vi "Test_ANN.vi"(8 "error in (no error)":errorcluster, 11 "FPGA VI Reference In":refnum<k20>) -> (0 "error out":errorcluster, 2 "Acc":dbl, 3 "FPGA VI Reference Out":refnum<k20>)   [LabVIEW 2020]
uses:
  <vilib>/Utility/error.llb/Error Cluster From Error Code.vi
  <vilib>/rvi/errors/niLvFpgaAdjustHostInterfaceError.vi
  Store Training and Testing set.vi
  <vilib>/rvi/interface/nirviMethod/nirviMethod.xnode
  <vilib>/FPGAPlugInAG/Dynamic/niLvFpga_WriteFifo_Dynamic.vi
  <vilib>/rvi/errors/niLvFpgaMergeErrorWithErrorCode.vi
  <vilib>/FPGAPlugInAG/Dynamic/niLvFpga_ReadFifo_Dynamic.vi
panel:
  out "Prediction":sgl[](array[numeric])
  out "Real":sgl[](array[numeric])
  out "good":i32
  out "total":i32
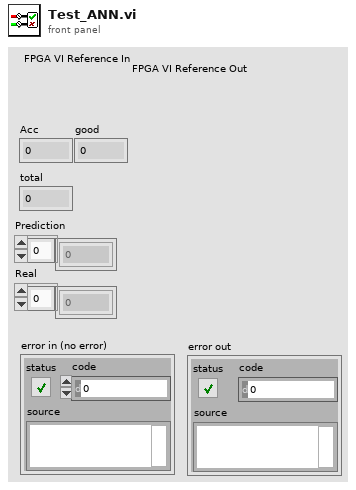
[diagram p1: front panel]
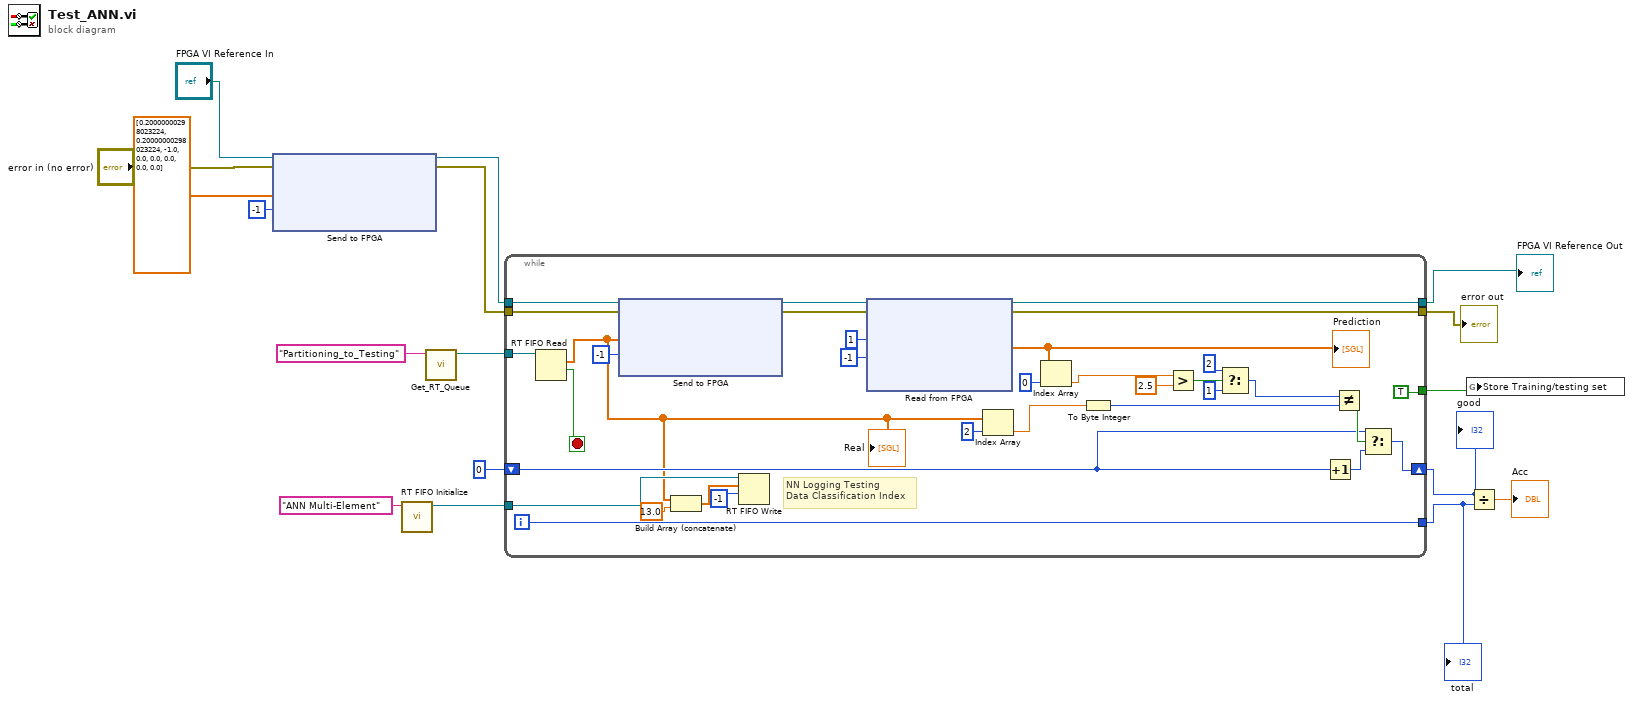
[diagram p0: block diagram]
diagram:
  n1 = xnode "Send to FPGA"("FPGA VI Reference In"="FPGA VI Reference In", "error in"="error in (no error)", "Data"=sgl[] [0.2, 0.2, -1.0, 0.0, 0.0, 0.0, 0.0, 0.0] ("Data to FPGA"), "Timeout (ms)"=-1) -> ("FPGA VI Reference Out"=w14:refnum<k20>, "error out"=w13:errorcluster)  [unwired: 1 out]
  n2 = call "RT FIFO Initialize.vi"("name (unnamed)"="ANN Multi-Element") -> ("rt fifo"=w4:refnum<k33>)  [unwired: 9 in, 1 out]
  n3 = call "Get_RT_Queue.vi"("String"="Partitioning_to_Testing") -> ("rt fifo single"=w6:refnum<k33>)  [unwired: 8 in, 2 out]
  n4 = while {
    tunnel: w14 -> [w49]
    tunnel: w13 -> [w48]
    tunnel: [w42] -> w1
    tunnel: [w41] -> w12
    shift-right: [w36] -> w10
    shift-left: 0 -> [w38]
    tunnel: [w40] -> w9
    tunnel: w6 -> [w33]
    tunnel: w4 -> [w20]
    tunnel: [TRUE] -> w3
    i -> [w40]
    stop <- w50 stop-if-true
    # "NN Logging Testing \nData Classification Index"
    n5 = RT FIFO Read(0:w33) -> (9:w19:sgl[], 10:w50:bool)  [unwired: 3 in, 3 out]
    "Real" <- w19
    n6 = xnode "Send to FPGA"("FPGA VI Reference In"=w49, "error in"=w48, "Data"=w19, "Timeout (ms)"=-1) -> ("FPGA VI Reference Out"=w47:refnum<k20>, "error out"=w46:errorcluster)  [unwired: 1 out]
    n7 = Build Array (concatenate)(w19, 13.0) -> (w23:dbl[])
    n8 = RT FIFO Write(0:w20, 1:w23, 2:-1 ("timeout in ms (0)")) -> ()  [unwired: 2 in, 4 out]
    n9 = xnode "Read from FPGA"("FPGA VI Reference In"=w47, "error in"=w46, "Number of Elements"=u32 1, "Timeout (ms)"=-1) -> ("FPGA VI Reference Out"=w42:refnum<k20>, "error out"=w41:errorcluster, "Data"=w44:sgl[])  [unwired: 1 out]
    "Prediction" <- w44
    n10 = Index Array(array=w19, index=2) -> (element=w31:sgl)
    n11 = Index Array(array=w44, index=0) -> (element=w29:sgl)
    n12 = To Byte Integer(number=w31) -> (8bit integer=w30:i8)
    n13 = Greater?(x=w29, y=sgl 2.5) -> (0:w27:bool)
    n14 = Select(t=i8 2, s=w27, f=i8 1) -> (s? t:f=w24:i8)
    n15 = Increment(x=w38) -> (x+1=w37:i32)
    n16 = Not Equal?(x=w24, y=w30) -> (x != y?=w39:bool)
    n17 = Select(t=w38, s=w39, f=w37) -> (s? t:f=w36:i32)
  }
  "error out" <- w12
  "total" <- w9
  "good" <- w10
  "FPGA VI Reference Out" <- w1
  n18 = global write "Store Training and Testing set.vi" "Store Training/testing set"(w3) -> ()
  n19 = Divide(x=w10, y=w9) -> (x/y=→"Acc":dbl)
